vi "Queue Monitor.vi"(11 "Queue Ref In":T1={"UI"=refnum, "Message"=refnum, "Data"=refnum, "Caller"=refnum, "Name"="000 Common", "Data Path"=path "", "Class Path"=path "", "SubPanel"=refnum, "Project Name"="", "MNT"="", "Title"="", "Data Source"=refnum, "Queue List"={}, "VI"=refnum, "UE"=refnum}) -> ()   [LabVIEW 2020]
doc: "Monitor"
uses:
  000 Module Data Type.ctl
  Queue Message.ctl
panel:
  out "Num":u32
  in  "Max Meesage Number":i32=100
  in  "Clear":bool
  out "Message":T2(array[cluster])
  in  "Search":string
  out "Count":u32
  out "Data List":string[][](table)
  out "Count0":u32 caption="Time Count"
  out "Elapsed time(ms)":u32
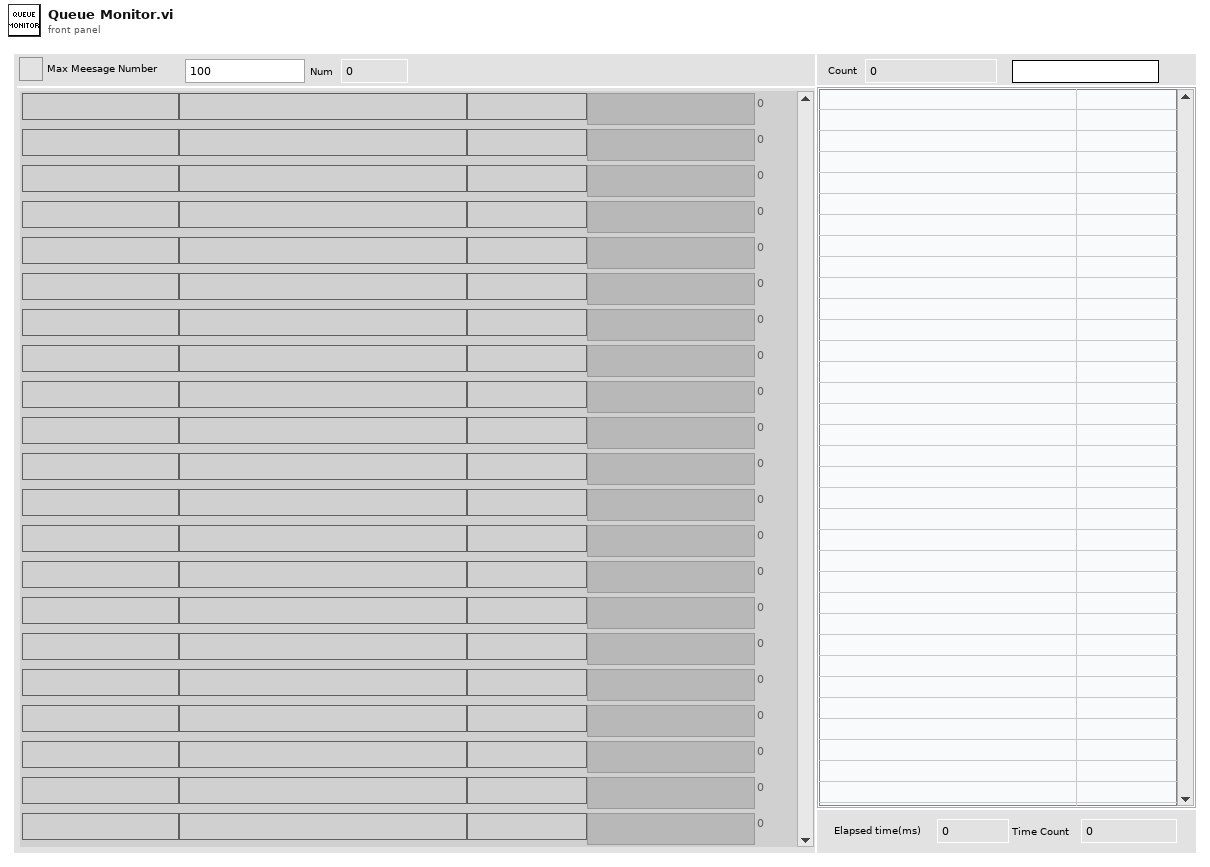
[diagram p1: front panel]
types:
  T1 = typedef "000 Module Data Type.ctl" = cluster{"UI":refnum<queue>, "Message":refnum<queue>, "Data":refnum<queue>, "Caller":refnum<queue>, "Name":string, "Data Path":path, "Class Path":path, "SubPanel":refnum<vi>, "Project Name":string, "MNT":string, "Title":string, "Data Source":refnum<queue>, "Queue List":map{string, refnum<queue>}, "VI":refnum<vi>, "UE":refnum<user-event>}
  T2 = cluster{"Time":string, "Name":string, "Message":string, "Data":variant, "elements":i32}[]
  T3 = cluster{"Time":string, "Name":string, "Message":string, "Data":variant, "elements":i32}
  T4 = cluster{"Message":cluster{"Time":string, "Name":string, "Message":string, "Data":variant, "elements":i32}[], "Delay":cluster{"Count Time(ms)":u32, "Delay Time(ms)":u32, "Next":string}}
  T5 = typedef "LVPoint32TypeDef.ctl" = cluster{"Horizontal":i32, "Vertical":i32}
  T6 = typedef "LVRowAndColumnTypeDef.ctl" = cluster{"Row":i32, "Column":i32}
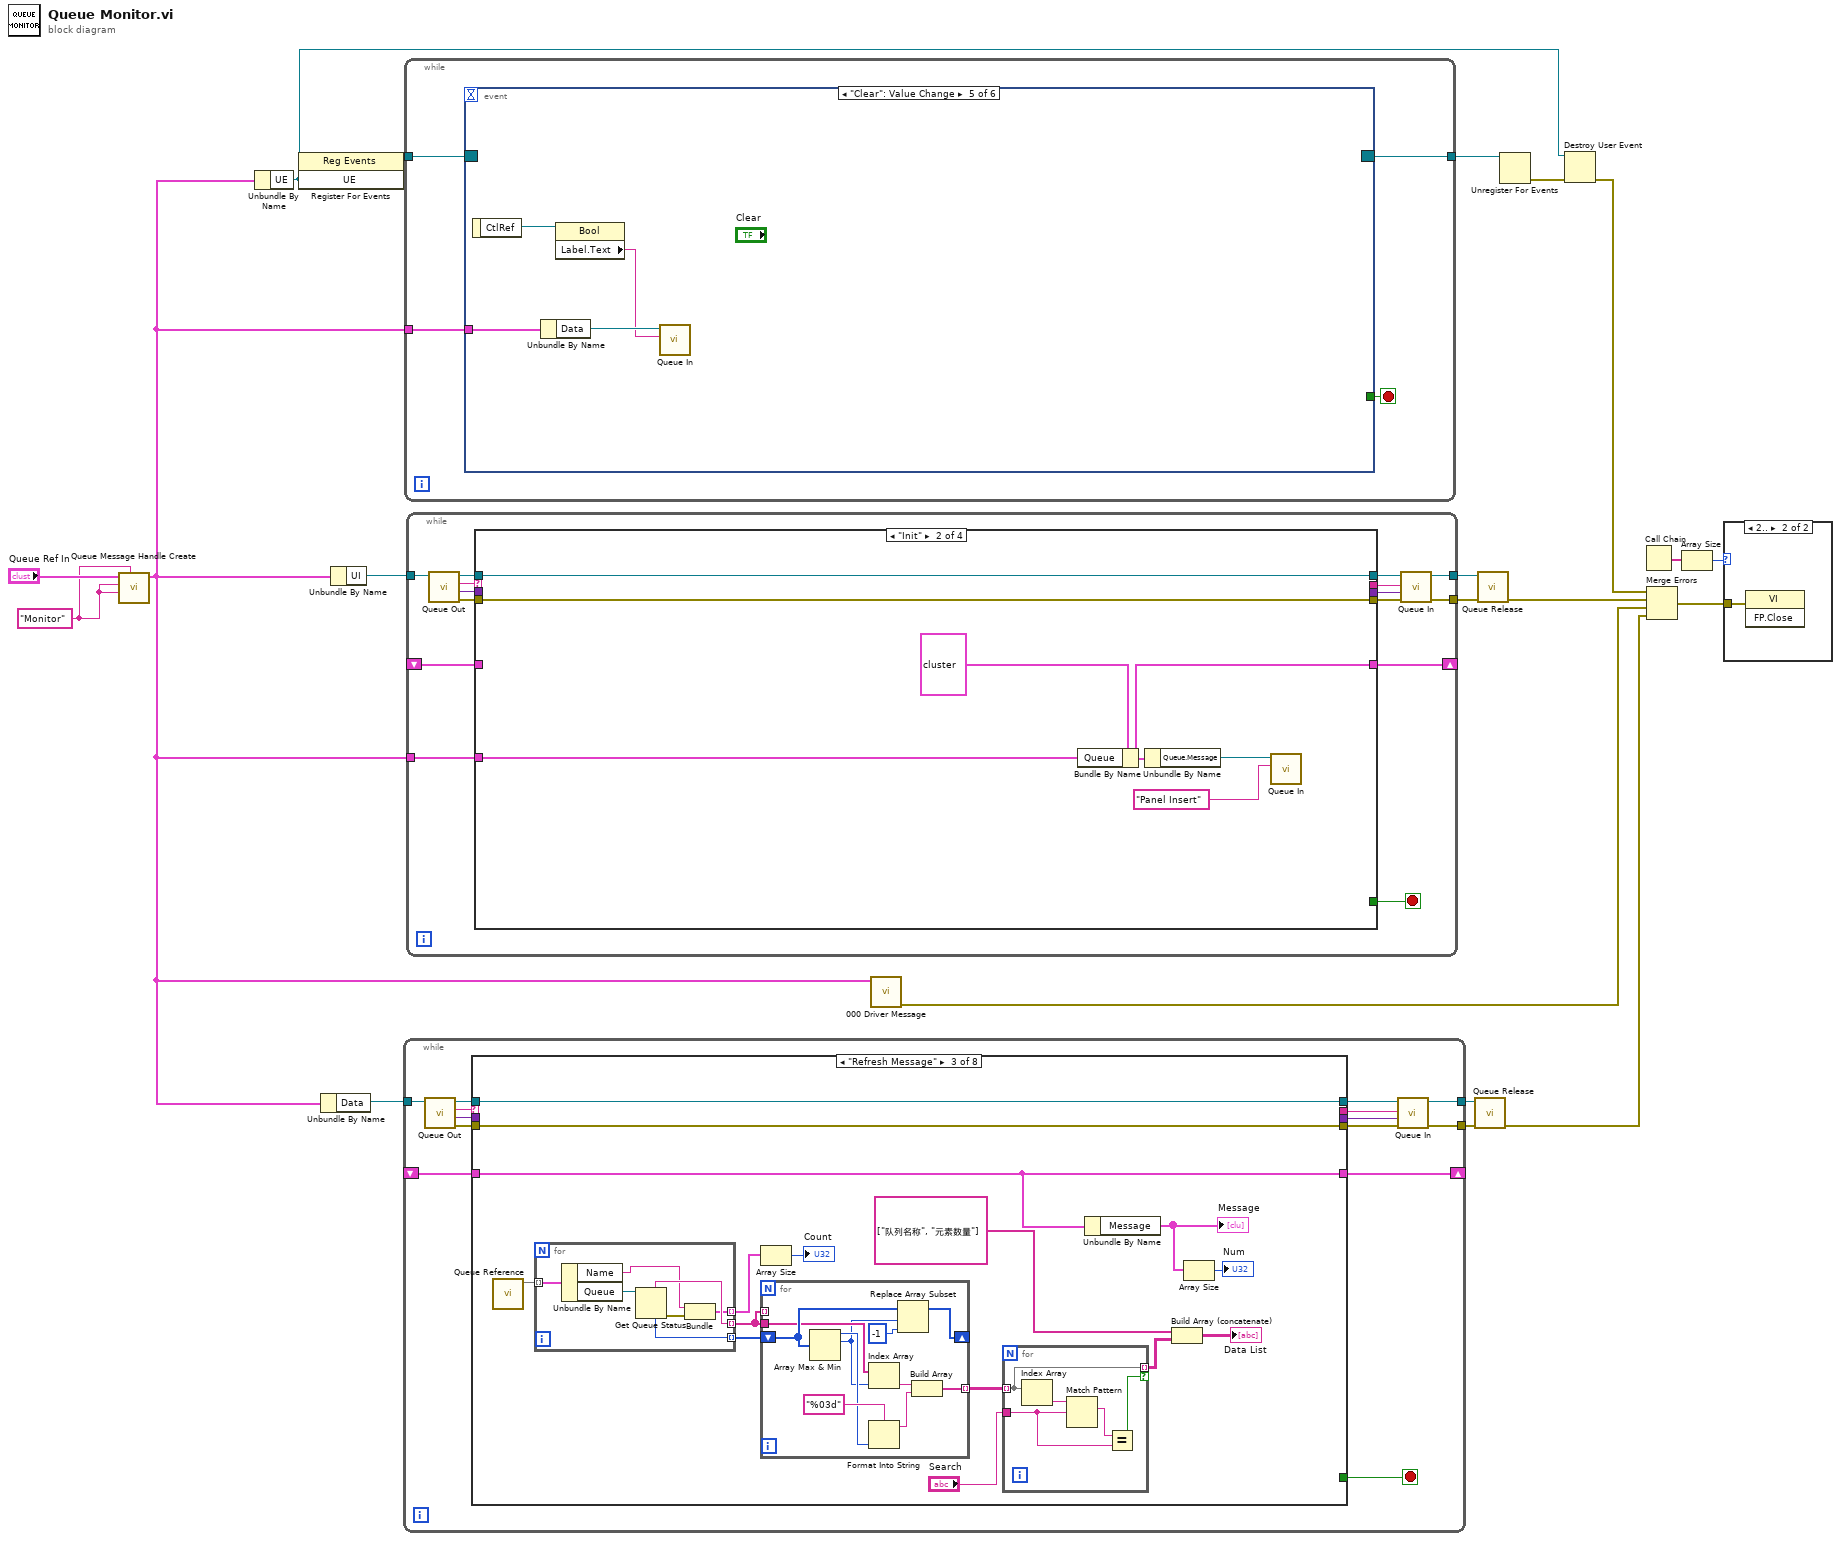
[diagram p0: block diagram]
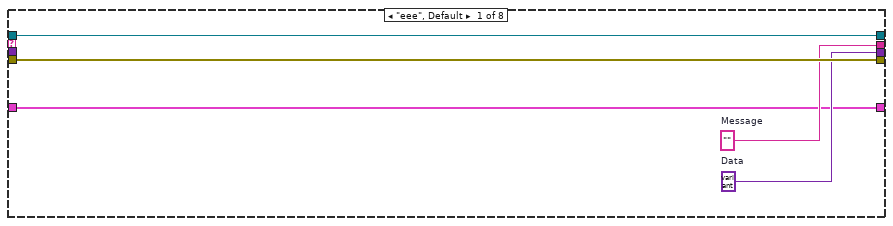
[diagram p2: hidden frame]
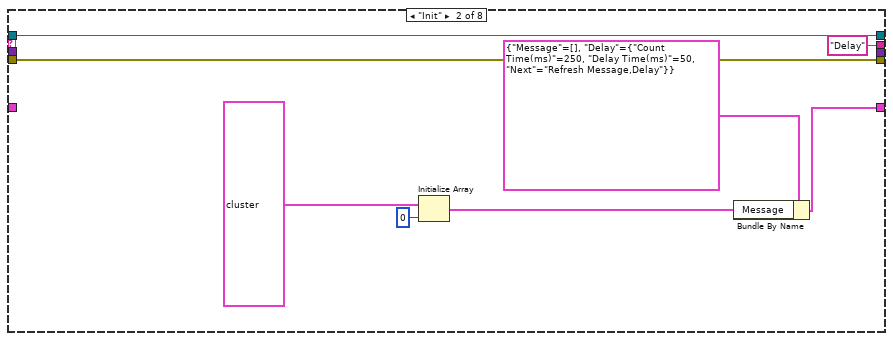
[diagram p3: hidden frame]
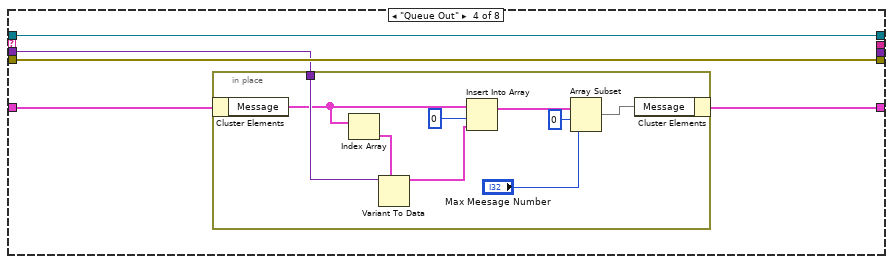
[diagram p4: hidden frame]
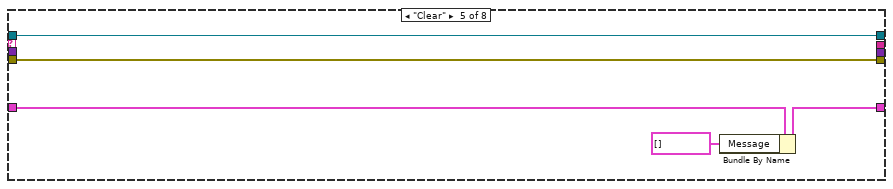
[diagram p5: hidden frame]
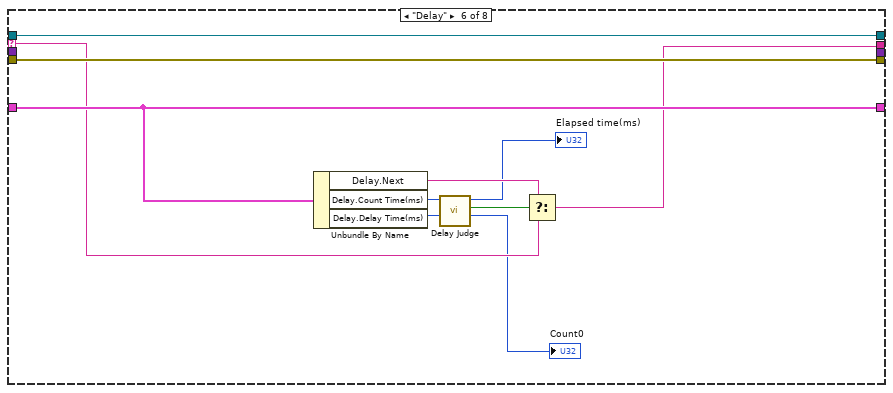
[diagram p6: hidden frame]
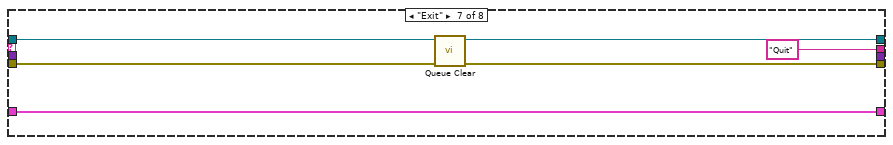
[diagram p7: hidden frame]
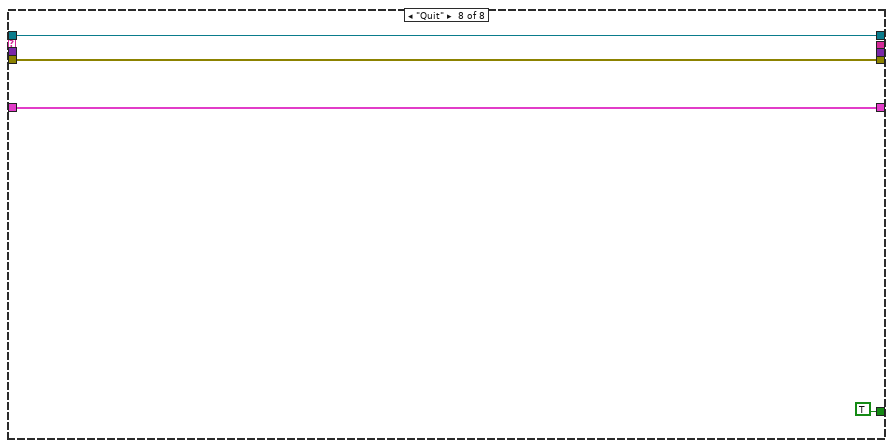
[diagram p8: hidden frame]
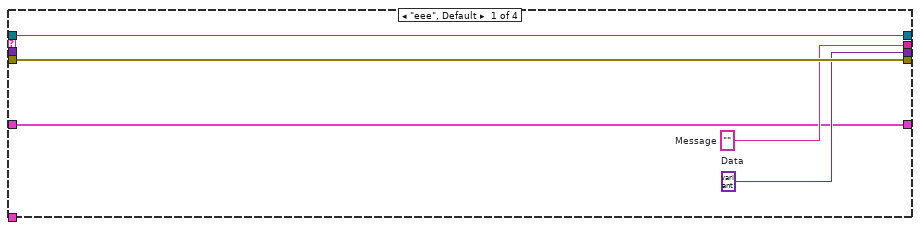
[diagram p10: hidden frame]
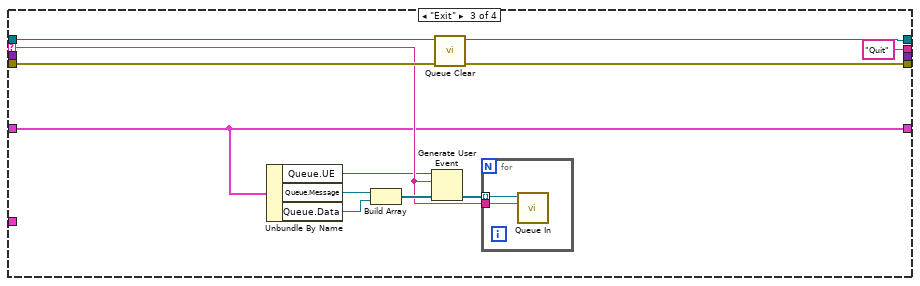
[diagram p11: hidden frame]
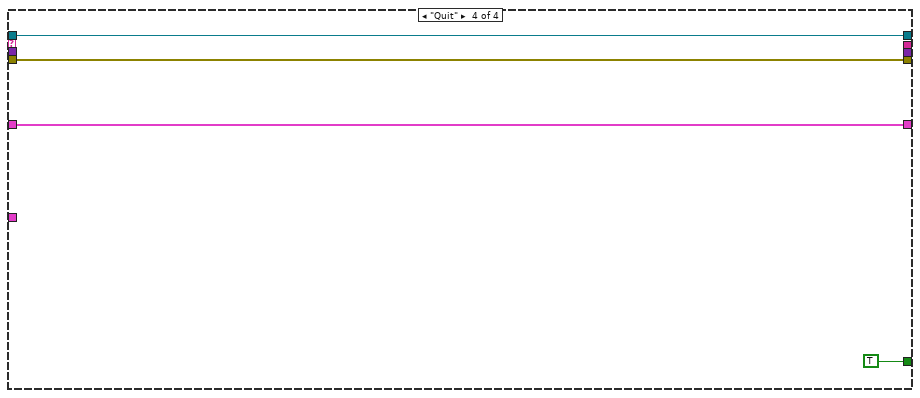
[diagram p12: hidden frame]
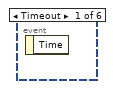
[diagram p13: hidden frame]
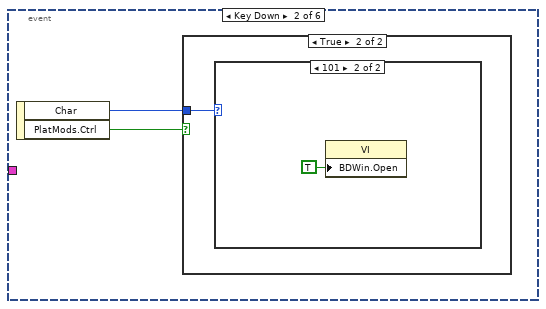
[diagram p14: hidden frame]
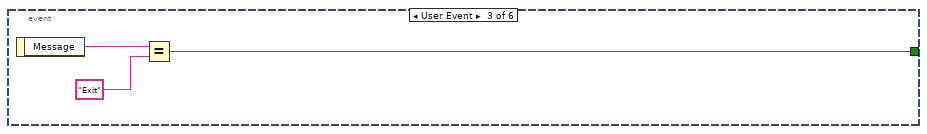
[diagram p17: hidden frame]
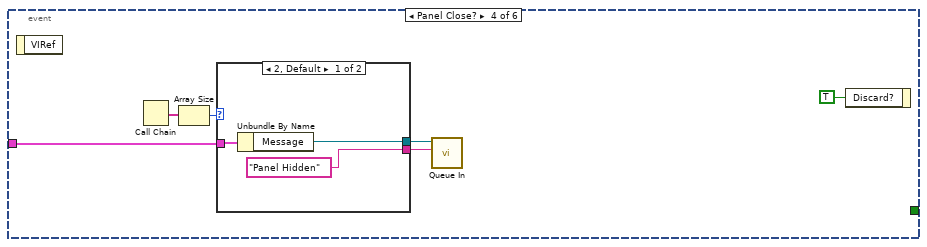
[diagram p18: hidden frame]
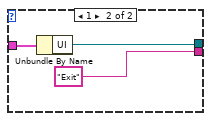
[diagram p19: hidden frame]
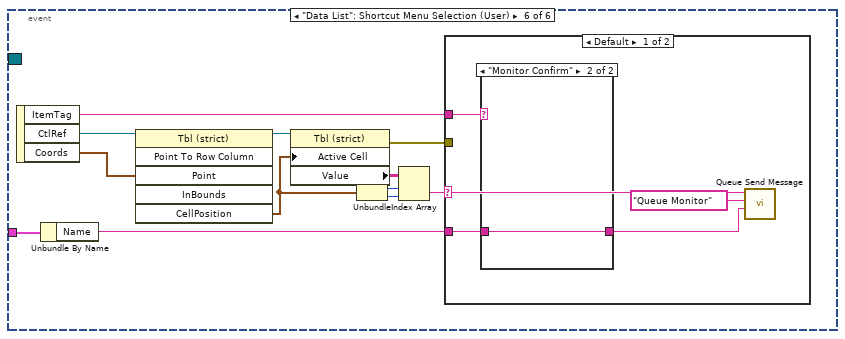
[diagram p20: hidden frame]
diagram:
  w1 = "Monitor" ("Name")
  n1 = call "Queue Message Handle Create.vi"("Project Name"=w1, "Name"=w1, "Title"=w1, "Queue Ref In"="Queue Ref In") -> ("Queue Ref Out"=w3:T1)  [unwired: 5 in, 2 out]
  n2 = Unbundle By Name(w3) -> ("UE"=w2:refnum<user-event>)
  n3 = register-events(w2) -> (reference out=w4:refnum<event-registration>)  [unwired: 2 in, 1 out]
  n4 = Unbundle By Name(w3) -> ("Data"=w17:refnum<queue>)
  n5 = Unbundle By Name(w3) -> ("UI"=w9:refnum<queue>)
  n6 = while {
    tunnel: w17 -> [w30]
    tunnel: [w27] -> w15
    tunnel: [w26] -> w16
    shift-right: [w21] -> _
    shift-left: _ -> [w22]
    stop <- w34 stop-if-true
    n7 = call "Queue Out.vi"("Queue In"=w30) -> ("error out"=w33:errorcluster, "Data"=w31:variant, "Message"=w32:string, "Queue Out"=w29:refnum<queue>)  [unwired: 6 in, 1 out]
    n8 = case shown="\"Refresh Message\"" w32 {
      selector: w32 -> [_ _ _ _ _ w107 _ _]
      tunnel: w29 -> [w39 w47 w62 w89 w103 w114 w119 w123]
      tunnel: w33 -> [w38 w46 w61 w88 w102 w113 w117 w124]
      tunnel: [w39 w47 w62 w89 w103 w114 w118 w123] -> w28
      tunnel: [w38 w46 w61 w88 w102 w113 w116 w124] -> w25
      tunnel: [w37 "Delay" ("Next") _ _ _ w106 "Quit" _] -> w24
      tunnel: [_ _ _ _ _ _ _ TRUE] -> w34
      tunnel: [w36 _ _ _ _ _ _ _] -> w23
      tunnel: w31 -> [_ _ _ w87 _ _ _ _]
      tunnel: [w35 w42 w60 w85 w100 w108 w115 w121] -> w21
      tunnel: w22 -> [w35 _ w60 w86 w101 w108 w115 w121]
      frame "eee", Default {
        w36 = variant  # Data
        w37 = ""  # Message
      }
      frame "Init" {
        n9 = Initialize Array(T3 {"Time"="", "Name"="", "Message"="", "Data"=variant, "elements"=0} ("Menu"), 0 ("维数大小")) -> (w43:T2)
        n10 = Bundle By Name(cluster=T4 {"Message"=[], "Delay"={"Count Time(ms)"=250, "Delay Time(ms)"=50, "Next"="Refresh Message,Delay"}}, "Message"=w43) -> (w42:T4)
      }
      frame "Refresh Message" {
        n11 = call "Queue Reference.vi"() -> ("All Queue"=w57:map{string, refnum<queue>})  [unwired: 8 in, 3 out]
        n12 = for {
          tunnel: w57 -> [w84] mode=indexing
          tunnel: [w82] -> w55 mode=indexing
          tunnel: [w81] -> w56 mode=indexing
          tunnel: [w78] -> w58 mode=indexing
          n13 = Unbundle By Name(w84) -> ("Name"=w79:string, "Queue"=w83:refnum<queue>)
          n14 = Get Queue Status(queue=w83) -> (queue name=w82:string, error out=w80:errorcluster, # elements in queue=w81:i32)  [unwired: 2 in, 5 out]
          n15 = Bundle("Name"=w79, "error out"=w80) -> (w78:cluster{"Name":string, "error out":errorcluster})  [unwired: 1 in]
        }
        n16 = Array Size(array=w58) -> (size(s)=→"Count":i32)
        n17 = for {
          shift-right: [w76] -> _
          shift-left: w56 -> [w77]
          tunnel: w55 -> [w75]
          tunnel: w55 -> [_] mode=indexing
          tunnel: [w68] -> w50 mode=indexing
          n18 = Array Max & Min(array=w77) -> (max value=w73:i32, max index (indices)=w70:i32)  [unwired: 2 out]
          n19 = Index Array(array=w75, index=w70) -> (element=w72:string)
          n20 = Format Into String(format string="%03d" ("格式字符串"), w73) -> (resulting string=w71:string)  [unwired: 2 in, 1 out]
          n21 = Replace Array Subset(array=w77, new element=-1 ("新元素/子数组"), index=w70) -> (w76:i32[])
          n22 = Build Array(w72, w71) -> (w68:string[])
        }
        n23 = for {
          tunnel: w50 -> [w64] mode=indexing
          tunnel: "Search" -> [w65]
          tunnel: [w64] -> w48 mode=indexing if=w63
          n24 = Index Array(array=w64) -> (element=w67:string)  [unwired: 1 in]
          n25 = Match Pattern(string=w67, regular expression=w65) -> (match substring=w66:string)  [unwired: 1 in, 3 out]
          n26 = Equal?(x=w66, y=w65) -> (x = y?=w63:bool)
        }
        n27 = Unbundle By Name(w60) -> ("Message"=w51:T2)
        "Message" <- w51
        n28 = Build Array (concatenate)(string[] ["队列名称", "元素数量"] ("列首字符串[]"), w48) -> (→"Data List":string[][])
        n29 = Array Size(array=w51) -> (size(s)=→"Num":i32)
      }
      frame "Queue Out" {
        n30 = in-place {
          in-place-border: w87 -> [w98]
          n31 = in-place-cluster #1(w86) -> ("Message"=w94:T2)
          n32 = Index Array(array=w94) -> (element=w95:T3)  [unwired: 1 in]
          n33 = Variant To Data(type=w95, Variant=w98) -> (data=w93:T3)  [unwired: 1 in, 1 out]
          n34 = Insert Into Array(array=w94, index=0 ("索引"), new element=w93) -> (w91:T2)
          n35 = Array Subset(array=w91, index=0 ("索引"), length="Max Meesage Number") -> (w90:T2)
          n36 = in-place-cluster #1("Message"=w90) -> (w85:T4)
        }
      }
      frame "Clear" {
        n37 = Bundle By Name(cluster=w101, "Message"=T2 []) -> (w100:T4)
      }
      frame "Delay" {
        n38 = Unbundle By Name(w108) -> ("Delay.Next"=w112:string, "Delay.Count Time(ms)"=w109:u32, "Delay.Delay Time(ms)"=w110:u32)
        n39 = call "Delay Judge.vi"("Delay Time(ms)"=w110, "Count Time(ms)"=w109) -> ("Count"=→"Count0":u32, "Time Out?"=w111:bool, "Elapsed time(ms)"=→"Elapsed time(ms)":u32)  [unwired: 5 in, 2 out]
        n40 = Select(t=w112, s=w111, f=w107) -> (s? t:f=w106:string)
      }
      frame "Exit" {
        n41 = call "Queue Clear.vi"("error in (no error)"=w117, "Queue In"=w119) -> ("error out"=w116:errorcluster, "Queue Out"=w118:refnum<queue>)  [unwired: 8 in]
      }
      frame "Quit" {
      }
    }
    n42 = call "Queue In.vi"("error in (no error)"=w25, "Data"=w23, "Message"=w24, "Queue In"=w28) -> ("error out"=w26:errorcluster, "Queue Out"=w27:refnum<queue>)  [unwired: 6 in]
  }
  n43 = while {
    tunnel: w4 -> [w128]
    tunnel: [w126] -> w5
    tunnel: w3 -> [w125]
    stop <- w127 stop-if-true
    n44 = event shown="[4] \"Clear\": Value Change" {
      selector: w128 -> [_ _ _ _ _ _]
      dyn-events: [_ _ _ _ _ _] -> w126
      timeout: _ -> [_ _ _ _ _ _]
      tunnel: [_ _ w133 _ _ _] -> w127
      tunnel: w125 -> [_ _ _ w138 w151 w163]
      event Timeout {
        n45 = event-data() -> ()  [unwired: 1 in, 1 out]
      }
      event Key Down {
        n46 = event-data() -> ("Char"=w130:i16, "PlatMods.Ctrl"=w129:bool)  [unwired: 1 in]
        n47 = case shown="True" w129 {
          tunnel: w130 -> [_ w131]
          frame False {
          }
          frame True {
            n48 = case shown="101" w131 {
              frame 0, Default {
              }
              frame 101 {
                n49 = property class="VI"("BDWin.Open"=TRUE ("程序框图窗口:打开")) -> ()  [unwired: 2 in, 2 out]
              }
            }
          }
        }
      }
      event User Event {
        n50 = event-data() -> ("Message"=w135:string)  [unwired: 1 in]
        n51 = Equal?(x=w135, y="Exit") -> (x = y?=w133:bool)
      }
      event Panel Close? {
        n52 = event-data() -> ()  [unwired: 1 in, 1 out]
        n53 = Call Chain() -> (call chain=w140:string[])
        n54 = Array Size(array=w140) -> (size(s)=w139:i32)
        n55 = case shown="2, Default" w139 {
          tunnel: w138 -> [w144 w147]
          tunnel: [w143 w146] -> w137
          tunnel: ["Panel Hidden" ("Message") "Exit" ("Message")] -> w136
          frame 2, Default {
            n56 = Unbundle By Name(w144) -> ("Message"=w143:refnum<queue>)
          }
          frame 1 {
            n57 = Unbundle By Name(w147) -> ("UI"=w146:refnum<queue>)
          }
        }
        n58 = call "Queue In.vi"("Message"=w136, "Queue In"=w137) -> ()  [unwired: 8 in, 2 out]
        n59 = event-data("Discard?"=TRUE ("放弃？")) -> ()  [unwired: 1 in, 1 out]
      }
      event "Clear": Value Change {
        n60 = event-data() -> ("CtlRef"=w150:refnum<vi>)  [unwired: 1 in]
        n61 = Unbundle By Name(w151) -> ("Data"=w149:refnum<queue>)
        n62 = property class="Bool"(reference=w150) -> ("Label.Text"=w148:string)  [unwired: 1 in, 2 out]
        n63 = call "Queue In.vi"("Message"=w148, "Queue In"=w149) -> ()  [unwired: 8 in, 2 out]
      }
      event "Data List": Shortcut Menu Selection (User) {
        n64 = event-data() -> ("ItemTag"=w155:string, "CtlRef"=w162:refnum<vi>, "Coords"=w161:T5)  [unwired: 1 in]
        n65 = Unbundle By Name(w163) -> ("Name"=w152:string)
        n66 = invoke class="Tbl (strict)" method="Point To Row Column"(reference=w162, "Point"=w161) -> (reference out=w160:refnum<vi>, "CellPosition"=w159:T6)  [unwired: 4 in, 4 out]
        n67 = property class="Tbl (strict)"(reference=w160, "Active Cell"=w159) -> (error out=w154:errorcluster, "Value"=w153:string[][])  [unwired: 1 in, 1 out]
        n68 = Unbundle(w159) -> ("Row"=w158:i32, "Column"=w157:i32)
        n69 = Index Array(array=w153, index (row)=w158, index (col)=w157) -> (element=w156:string)
        n70 = case shown="Default" w156 {
          selector: w156 -> [w168 _]
          tunnel: w155 -> [w166 _]
          tunnel: w154 -> [_ _]
          tunnel: w152 -> [w165 _]
          frame Default {
            n71 = case shown="\"Monitor Confirm\"" w166 {
              tunnel: w165 -> [_ w169]
              tunnel: [_ w169] -> w164
              frame Default {
              }
              frame "Monitor Confirm" {
              }
            }
            n72 = call "Queue Send Message.vi"("Data"=w164, "Message"="Queue Monitor", "Queue Name"=w168) -> ()  [unwired: 6 in, 3 out]
          }
          frame "" {
          }
        }
      }
    }
  }
  n73 = while {
    tunnel: w9 -> [w180]
    tunnel: [w177] -> w7
    tunnel: [w176] -> w8
    tunnel: w3 -> [w172]
    shift-right: [w171] -> _
    shift-left: _ -> [w170]
    stop <- w184 stop-if-true
    n74 = call "Queue Out.vi"("Queue In"=w180) -> ("error out"=w183:errorcluster, "Data"=w181:variant, "Message"=w182:string, "Queue Out"=w179:refnum<queue>)  [unwired: 6 in, 1 out]
    n75 = case shown="\"Init\"" w182 {
      selector: w182 -> [_ _ w199 _]
      tunnel: w179 -> [w189 w196 w206 w212]
      tunnel: w183 -> [w188 w195 w204 w213]
      tunnel: [w189 w196 w205 w212] -> w178
      tunnel: [w188 w195 w203 w213] -> w175
      tunnel: [w187 _ "Quit" _] -> w174
      tunnel: [_ _ _ TRUE] -> w184
      tunnel: [w186 _ _ _] -> w173
      tunnel: w181 -> [_ _ _ _]
      tunnel: w172 -> [_ w193 _ _]
      tunnel: [w185 w192 w198 w210] -> w171
      tunnel: w170 -> [w185 _ w198 w210]
      frame "eee", Default {
        w186 = variant  # Data
        w187 = ""  # Message
      }
      frame "Init" {
        n76 = Bundle By Name(cluster=cluster{"Queue":T1} {"Queue"={"UI"=refnum, "Message"=refnum, "Data"=refnum, "Caller"=refnum, "Name"="000 Common", "Data Path"=path "", "Class Path"=path "", "SubPanel"=refnum, "Project Name"="", "MNT"="", "Title"="", "Data Source"=refnum, "Queue List"={}, "VI"=refnum, "UE"=refnum}}, "Queue"=w193) -> (w192:cluster{"Queue":T1})
        n77 = Unbundle By Name(w192) -> ("Queue.Message"=w191:refnum<queue>)
        n78 = call "Queue In.vi"("Message"="Panel Insert", "Queue In"=w191) -> ()  [unwired: 8 in, 2 out]
      }
      frame "Exit" {
        n79 = Unbundle By Name(w198) -> ("Queue.UE"=w197:refnum<user-event>, "Queue.Message"=w202:refnum<queue>, "Queue.Data"=w201:refnum<queue>)
        n80 = Build Array(w202, w201) -> (w200:refnum<queue>[])
        n81 = Generate User Event(user event=w197, event data cluster=w199) -> ()  [unwired: 2 in, 2 out]
        n82 = call "Queue Clear.vi"("error in (no error)"=w204, "Queue In"=w206) -> ("error out"=w203:errorcluster, "Queue Out"=w205:refnum<queue>)  [unwired: 8 in]
        n83 = for {
          tunnel: w200 -> [w209] mode=indexing
          tunnel: w199 -> [w208]
          n84 = call "Queue In.vi"("Message"=w208, "Queue In"=w209) -> ()  [unwired: 8 in, 2 out]
        }
      }
      frame "Quit" {
      }
    }
    n85 = call "Queue In.vi"("error in (no error)"=w175, "Data"=w173, "Message"=w174, "Queue In"=w178) -> ("error out"=w176:errorcluster, "Queue Out"=w177:refnum<queue>)  [unwired: 6 in]
  }
  n86 = call "000 Driver Message.vi"("Queue In"=w3) -> ("error out"=w19:errorcluster)  [unwired: 8 in, 2 out]
  n87 = call "Queue Release.vi"("error in (no error)"=w16, "Queue In"=w15) -> ("error out"=w18:errorcluster)  [unwired: 9 in]
  n88 = call "Queue Release.vi"("error in (no error)"=w8, "Queue In"=w7) -> ("error out"=w11:errorcluster)  [unwired: 9 in]
  n89 = Unregister For Events(event registration refnum=w5) -> (error out=w6:errorcluster)  [unwired: 1 in]
  n90 = Destroy User Event(user event=w2, error in=w6) -> (error out=w10:errorcluster)
  n91 = Call Chain() -> (call chain=w13:string[])
  n92 = Merge Errors(w10, w11, w19, w18) -> (w12:errorcluster)
  n93 = Array Size(array=w13) -> (size(s)=w14:i32)
  n94 = case shown="2.." w14 {
    tunnel: w12 -> [_ w214]
    frame 0, Default {
    }
    frame 2.. {
      n95 = invoke class="VI" method="FP.Close"(error in=w214) -> ()  [unwired: 2 in, 3 out]
    }
  }
